vi "hp83623a_close_all.vi"(8 "error in":errorcluster, 11 "HP83623A Generator Settings Array":T1) -> (0 "error out":errorcluster)   [LabVIEW 2013, in "HP83623A_RF_Generator.lvclass"]
uses:
  HP83623A_RF_Generator.lvclass
  HP83623A_array.ctl
  HP83623A.ctl
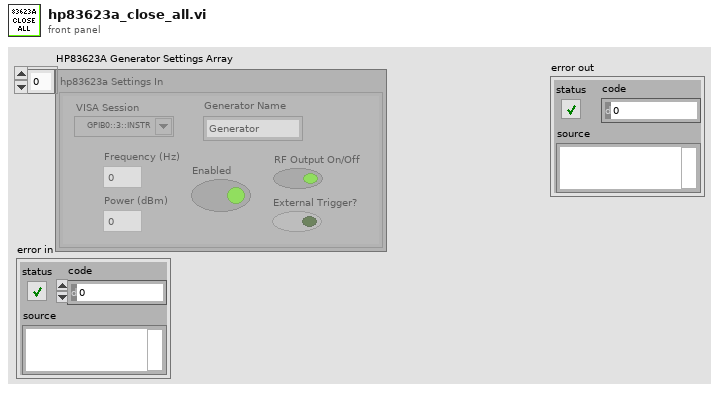
[diagram p1: front panel]
types:
  T1 = typedef "HP83623A_RF_Generator.lvclass/HP83623A_array.ctl" = T2[]
  T2 = typedef "HP83623A_RF_Generator.lvclass/HP83623A.ctl" = cluster{"Frequency (Hz)":dbl, "Power (dBm)":dbl, "Enabled":bool, "initialized":bool, "RF Output On/Off":bool, "External Trigger?":bool, "VISA Session":refnum<visa-resource-name>, "Generator Name":string}
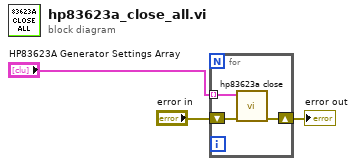
[diagram p0: block diagram]
diagram:
  n1 = for {
    tunnel: "HP83623A Generator Settings Array" -> [w4] mode=indexing
    shift-right: [w5] -> w1
    shift-left: "error in" -> [w6]
    n2 = call "hp83623a close.vi"("error in (no error)"=w6, "hp83623a Settings (in)"=w4) -> ("error out"=w5:errorcluster)  [unwired: 9 in]
  }
  "error out" <- w1
